vi "禹山pH_获取温度和测量值.vi"(8 "error in (no error)":errorcluster caption="错误输入（无错误）", 11 "MB session in":refnum<class "MB_Master.lvclass">) -> (0 "error out":errorcluster caption="错误输出", 2 "输出值":cluster{"温度测量值":sgl, "ORP":sgl, "pH":sgl}, 3 "MB session out":refnum<class "MB_Master.lvclass">)   [LabVIEW 2022 SP3, in "斯坦道多参数.lvlib"]
uses:
  <vilib>/Plasmionique/MB Master/MB_Master/MB_Master.lvclass
  <vilib>/Plasmionique/MB Master/MB Master.lvlib
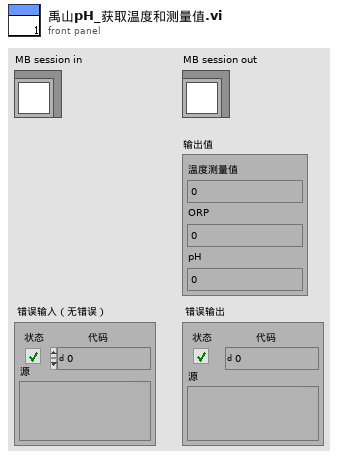
[diagram p1: front panel]
types:
  T1 = cluster{"pH":u32, "DO":u32, "Cond":u32, "Turb":u32, "叶绿素a":u32, "藻密度":u32, "ORP":u32, "COD":u32, "氯化物":u32, "氨氮":u32, "水中油":u32, "悬浮物":u32, "余氯":u32}
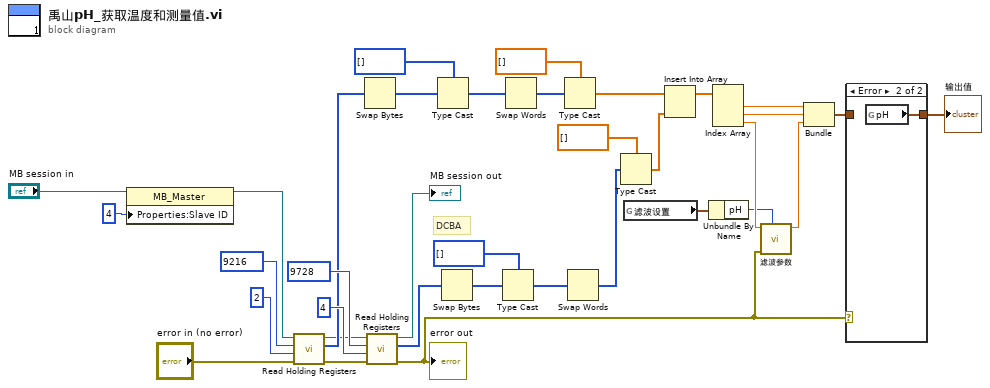
[diagram p0: block diagram]
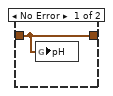
[diagram p2: hidden frame]
diagram:
  # "DCBA"
  n1 = property class="MB_Master"(reference="MB session in", "Properties:Slave ID"=u16 4 ("y")) -> (reference out=w13:refnum<class "MB_Master.lvclass">)  [unwired: 1 in, 1 out]
  n2 = call <vilib>:"Read Holding Registers.vi"("error in (no error)"="error in (no error)", "quantity"=u16 2, "starting address"=u16 9216, "MB session in"=w13) -> ("error out"=w14:errorcluster, "Registers"=w16:u16[], "MB session out"=w12:refnum<class "MB_Master.lvclass">)  [unwired: 5 in]
  n3 = Swap Bytes(anything=w16) -> (byte swapped=w21:u16[])
  n4 = call <vilib>:"Read Holding Registers.vi"("error in (no error)"=w14, "quantity"=u16 4, "starting address"=u16 9728, "MB session in"=w12) -> ("error out"=w1:errorcluster, "Registers"=w28:u16[], "MB session out"=→"MB session out":refnum<class "MB_Master.lvclass">)  [unwired: 5 in]
  "error out" <- w1
  n5 = Type Cast(type=u32[] [] ("数组 2"), x=w21) -> (*(type *) &x=w19:u32[])
  n6 = Swap Bytes(anything=w28) -> (byte swapped=w27:u16[])
  n7 = Type Cast(type=u32[] [] ("数组 2"), x=w27) -> (*(type *) &x=w31:u32[])
  n8 = Swap Words(1:w19) -> (0:w17:u32[])
  n9 = Type Cast(type=sgl[] [] ("数组 2"), x=w17) -> (*(type *) &x=w11:sgl[])
  n10 = Swap Words(1:w31) -> (0:w33:u32[])
  n11 = Type Cast(type=sgl[] [] ("数组 2"), x=w33) -> (*(type *) &x=w9:sgl[])
  n12 = global read "断电保存变量.vi" "滤波设置"() -> (w4:T1)
  n13 = Insert Into Array(array=w11, new element=w9) -> (w10:sgl[])  [unwired: 1 in]
  n14 = Unbundle By Name(w4) -> ("pH"=w3:u32)
  n15 = Index Array(array=w10) -> (element #1=w26:sgl, element #2=w25:sgl, element #3=w6:sgl)  [unwired: 3 in]
  n16 = call "滤波参数.vi"("滤波次数"=w3, "error in (no error)"=w1, "x"=w6) -> ("mode"=w5:dbl)  [unwired: 7 in, 1 out]
  n17 = Bundle("数值"=w26, "数值"=w25, "mode"=w5) -> (w24:cluster{"数值":sgl, "数值":sgl, "mode":dbl})  [unwired: 1 in]
  n18 = case shown="Error" w1 {
    tunnel: w24 -> [w36 _]
    tunnel: [w36 w37] -> w2
    frame No Error {
      n19 = global write "禹山过程全局变量.vi" "pH"(w36) -> ()
    }
    frame Error {
      n20 = global read "禹山过程全局变量.vi" "pH"() -> (w37:cluster{"温度测量值":sgl, "ORP":sgl, "pH":sgl})
    }
  }
  "输出值" <- w2
